vi "F1InfIn_Client_LabVIEW_Fita1.vi"() -> ()   [LabVIEW 2014]
panel:
  in  "IP":string
  in  "Pont":dbl
  in  "?":bool
  out "'X'":T1
  out "'U'":T2
  out "Resposta  \"Marxa / Parar\"":string
  out "'B'":T3
  in  "Port":dbl
  in  "IP":string
  out "Resposta  \"Reset mostra màxima i mínima\"":string
  out "'Y'":T4
  out "Tempreatura més antiga":dbl(graph)
  in  "Mensaje a enviar:":string(combo)
  in  "Numero de mostres":dbl
  in  "v":bool
  in  "Temps":dbl
  in  "?":bool
  # "GRUP -- A"
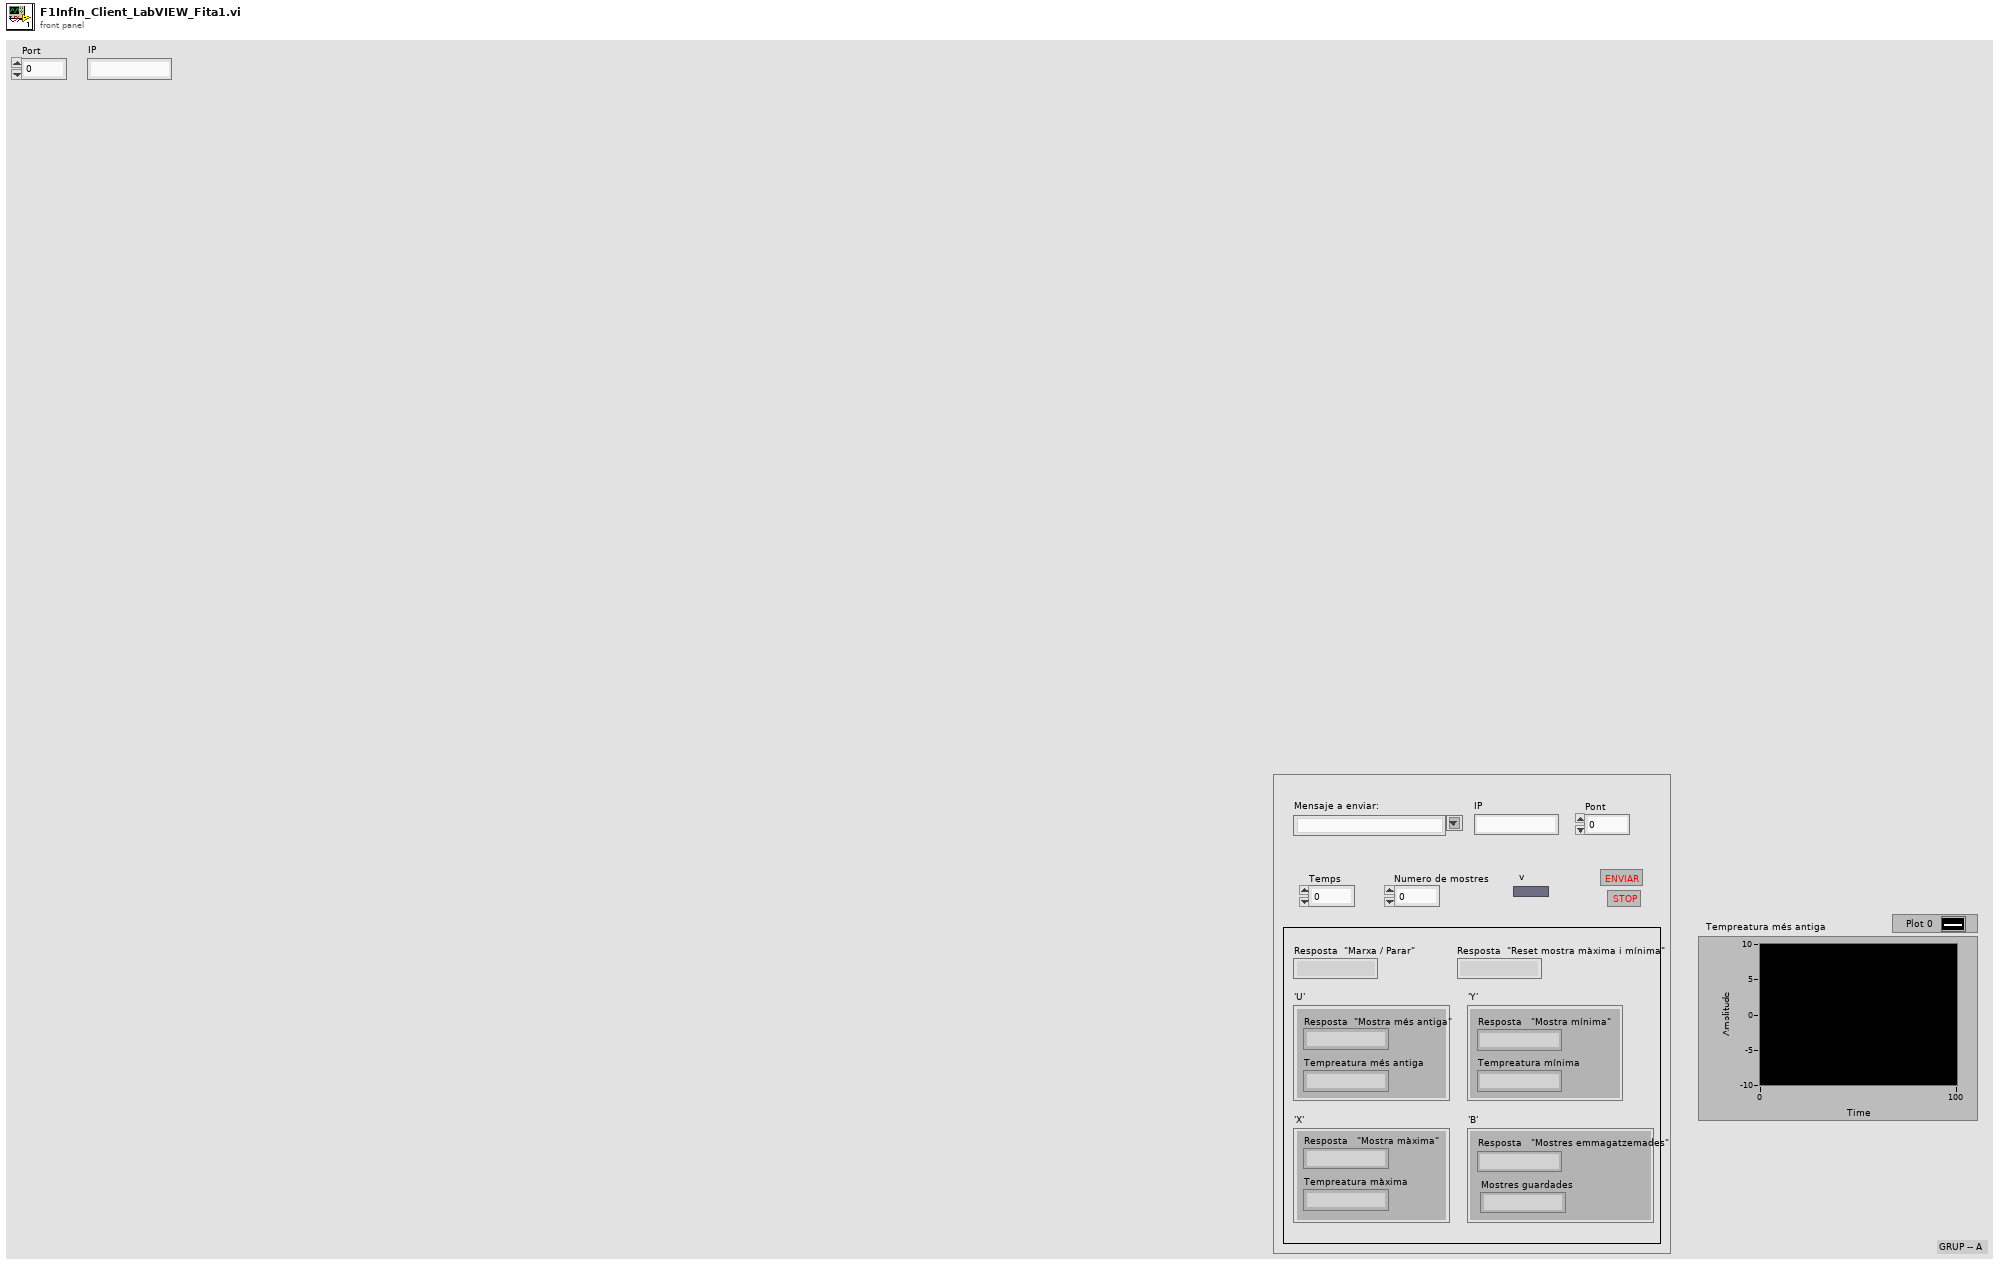
[diagram p1: front panel]
types:
  T1 = cluster{"Resposta   \"Mostra màxima\" ":string, "Tempreatura màxima":string}
  T2 = cluster{"Resposta  \"Mostra més antiga\" ":string, "Tempreatura més antiga":string}
  T3 = cluster{"Resposta   \"Mostres emmagatzemades\" ":string, "Mostres guardades ":string}
  T4 = cluster{"Resposta   \"Mostra mínima\"":string, "Tempreatura mínima":string}
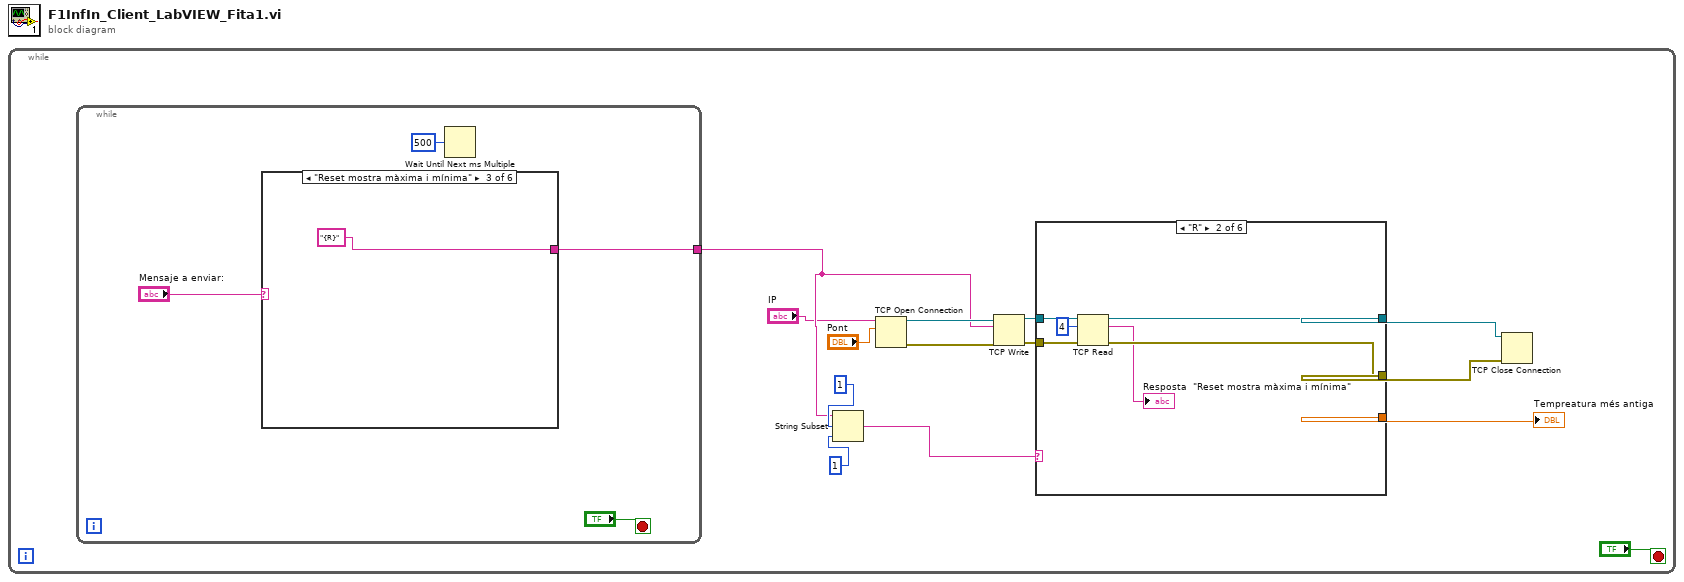
[diagram p0: block diagram]
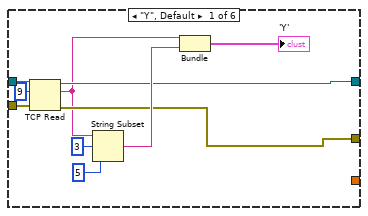
[diagram p2: hidden frame]
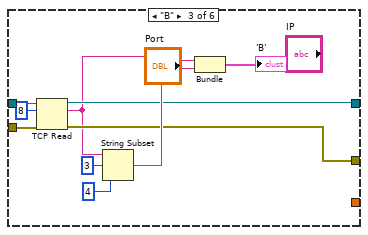
[diagram p3: hidden frame]
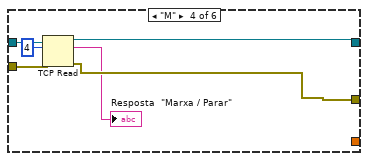
[diagram p4: hidden frame]
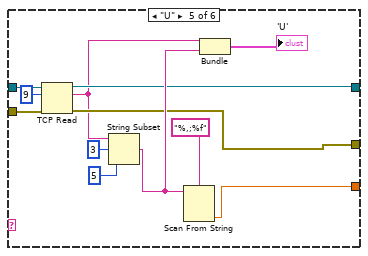
[diagram p5: hidden frame]
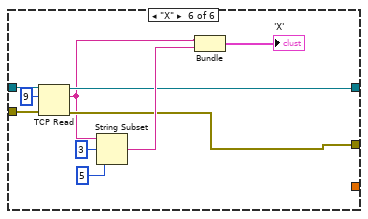
[diagram p6: hidden frame]
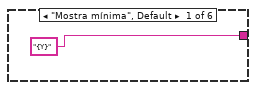
[diagram p7: hidden frame]
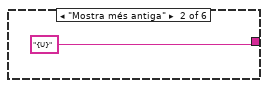
[diagram p8: hidden frame]
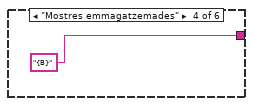
[diagram p9: hidden frame]
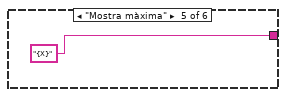
[diagram p10: hidden frame]
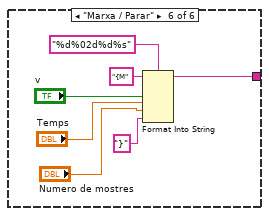
[diagram p11: hidden frame]
diagram:
  n1 = while {
    stop <- "?" stop-if-true
    n2 = while {
      tunnel: [w70] -> w4
      stop <- "?" stop-if-true
      n3 = case shown="\"Reset mostra màxima i mínima\"" "Mensaje a enviar:" {
        tunnel: ["{Y}" ("initial string") "{U}" ("initial string") "{R}" ("initial string") "{B}" ("initial string") "{X}" ("initial string") w78] -> w70
        frame "Mostra mínima", Default {
        }
        frame "Mostra més antiga" {
        }
        frame "Reset mostra màxima i mínima" {
        }
        frame "Mostres emmagatzemades" {
        }
        frame "Mostra màxima" {
        }
        frame "Marxa / Parar" {
          n4 = Format Into String(format string="%d%02d%d%s", initial string="{M", "v", "Temps", "Numero de mostres", "}" ("initial string")) -> (resulting string=w78:string)  [unwired: 1 in, 1 out]
        }
      }
      n5 = Wait Until Next ms Multiple(millisecond multiple=u32 500) -> ()  [unwired: 1 out]
    }
    n6 = String Subset(string=w4, offset (0)=1 ("length (rest)"), length (rest)=1 ("offset (0)")) -> (substring=w8:string)
    n7 = TCP Open Connection(address="IP", remote port or service name="Pont") -> (connection ID=w12:refnum<k5>, error out=w11:errorcluster)  [unwired: 3 in]
    n8 = TCP Write(connection ID=w12, data in=w4, error in (no error)=w11) -> (connection ID out=w14:refnum<k5>, error out=w13:errorcluster)  [unwired: 1 in, 1 out]
    n9 = case shown="\"R\"" w8 {
      tunnel: [w17 w28 w36 w43 w50 w62] -> w7
      tunnel: [w18 w27 w35 w44 w49 w61] -> w6
      tunnel: [_ _ _ _ w55 _] -> w5
      tunnel: w14 -> [w20 w30 w33 w46 w52 w64]
      tunnel: w13 -> [w19 w29 w32 w45 w51 w63]
      frame "Y", Default {
        n10 = TCP Read(connection ID=w20, bytes to read=9, error in (no error)=w19) -> (connection ID out=w17:refnum<k5>, data out=w16:string, error out=w18:errorcluster)  [unwired: 2 in]
        n11 = String Subset(string=w16, offset (0)=3, length (rest)=5 ("length (rest)")) -> (substring=w22:string)
        n12 = Bundle("data out"=w16, "data out"=w22) -> (→"'Y'":cluster{"data out":string, "data out":string})  [unwired: 1 in]
      }
      frame "R" {
        n13 = TCP Read(connection ID=w30, bytes to read=4, error in (no error)=w29) -> (connection ID out=w28:refnum<k5>, data out=→"Resposta  \"Reset mostra màxima i mínima\"":string, error out=w27:errorcluster)  [unwired: 2 in]
      }
      frame "B" {
        n14 = TCP Read(connection ID=w33, bytes to read=8, error in (no error)=w32) -> (connection ID out=w36:refnum<k5>, data out=w34:string, error out=w35:errorcluster)  [unwired: 2 in]
        n15 = String Subset(string=w34, offset (0)=3, length (rest)=4 ("length (rest)")) -> (substring=w37:string)
        n16 = Bundle("data out"=w34, "data out"=w37) -> (→"'B'":cluster{"data out":string, "data out":string})  [unwired: 1 in]
      }
      frame "M" {
        n17 = TCP Read(connection ID=w46, bytes to read=4, error in (no error)=w45) -> (connection ID out=w43:refnum<k5>, data out=→"Resposta  \"Marxa / Parar\"":string, error out=w44:errorcluster)  [unwired: 2 in]
      }
      frame "U" {
        n18 = TCP Read(connection ID=w52, bytes to read=9, error in (no error)=w51) -> (connection ID out=w50:refnum<k5>, data out=w48:string, error out=w49:errorcluster)  [unwired: 2 in]
        n19 = String Subset(string=w48, offset (0)=3, length (rest)=5 ("length (rest)")) -> (substring=w53:string)
        n20 = Scan From String(format string="%,;%f", input string=w53) -> (output 1=w55:dbl)  [unwired: 3 in, 3 out]
        n21 = Bundle("data out"=w48, "data out"=w53) -> (→"'U'":cluster{"data out":string, "data out":string})  [unwired: 1 in]
      }
      frame "X" {
        n22 = TCP Read(connection ID=w64, bytes to read=9, error in (no error)=w63) -> (connection ID out=w62:refnum<k5>, data out=w60:string, error out=w61:errorcluster)  [unwired: 2 in]
        n23 = String Subset(string=w60, offset (0)=3, length (rest)=5 ("length (rest)")) -> (substring=w65:string)
        n24 = Bundle("data out"=w60, "data out"=w65) -> (→"'X'":cluster{"data out":string, "data out":string})  [unwired: 1 in]
      }
    }
    "Tempreatura més antiga" <- w5
    n25 = TCP Close Connection(connection ID=w7, error in (no error)=w6) -> ()  [unwired: 1 in, 2 out]
  }
